vi "experiment control.vi"() -> ()   [LabVIEW 2012] (continued)
              tunnel: [w3762 w3766 w3770 w3775] -> w3734
              frame "A", Default {
                n1646 = Replace Array Subset(array=w3762, new element=TRUE ("new element/subarray"), index=w3765) -> (w3763:bool[])
              }
              frame "B" {
                n1647 = Replace Array Subset(array=w3766, new element=TRUE ("new element/subarray"), index=w3769) -> (w3767:bool[])
              }
              frame "C" {
                n1648 = Replace Array Subset(array=w3770, new element=TRUE ("new element/subarray"), index=w3773) -> (w3771:bool[])
              }
              frame "D" {
                n1649 = Replace Array Subset(array=w3774, new element=TRUE ("new element/subarray"), index=w3777) -> (w3775:bool[])
              }
            }
            n1650 = Bundle("Begin (ms)"=0.0, "Begin (ms)"=w3747, "DIO64 Line 4"=w3738, "DIO64 Line 4"=w3738, "DIO64 Line 4"=w3738, "DIO64 Line 4"=w3738) -> (w3749:T107)  [unwired: 1 in]
            n1651 = Bundle("Begin (ms)"=w3747, "Begin (ms)"=w3747, "DIO64 Line 4"=w3737, "DIO64 Line 4"=w3736, "DIO64 Line 4"=w3735, "DIO64 Line 4"=w3734) -> (w3752:T107)  [unwired: 1 in]
            n1652 = Bundle("Begin (ms)"=20.0, "Begin (ms)"=w3747, "DIO64 Line 4"=w3738, "DIO64 Line 4"=w3738, "DIO64 Line 4"=w3738, "DIO64 Line 4"=w3738) -> (w3748:T107)  [unwired: 1 in]
            n1653 = Build Array(w3749, w3752, w3748) -> (w3753:T108)
            n1654 = call "dt_i to 0-t_i.vi"("DIO64 Debug"=w3753) -> ("output cluster"=w3755:cluster{bool[][], bool[][], bool[][], bool[][]}, "DIOArray out 1"=w3756:bool[][], "ti"=w3757:dbl[])  [unwired: 2 in]
            n1655 = call "DIO64 Sequence.vi"("DIO64Addr (0)"=u16 0, "RepRate (Hz)"=10000.0, "Time Array (ms)"=w3757, "Set DIO line .."=w3756, "output cluster"=w3755, "error in"=w3760) -> ("error out"=w3759:errorcluster)  [unwired: 9 in]
          }
          frame "DIO64: Close" {
            n1656 = call "DIO64 Close.vi"("board in"=u16 0, "error in (no error)"=w3782) -> ("error out"=w3781:errorcluster)  [unwired: 12 in, 1 out]
            n1657 = Enqueue Element At Opposite End(queue=w3778, element="Debug: Console >> Closing DIO64") -> ()  [unwired: 2 in, 3 out]
          }
          frame "---------- Scope ----------" {
            # "Template Separator\n(You can make a copy of, or modify, this frame)"
          }
          frame "Scope: Initialise" {
            n1658 = case shown="\"TDS5034B\", Default" w3808 {
              tunnel: [w3812 w3814] -> w3795
              tunnel: ["SELect:CH4 ON" ("string") _] -> w3793
              tunnel: [w3812 w3814] -> w3791
              frame "TDS5034B", Default {
                n1659 = local read "TDS5034B Oscilloscope"() -> (w3812:T24)
              }
              frame "TDS2014" {
                n1660 = local read "TDS2014 Oscilloscope"() -> (w3814:T24)
              }
            }
            n1661 = Unbundle By Name(w3795) -> ("GPIB Address"=w3794:refnum<visa-resource-name>)
            n1662 = VISA Write(VISA resource name=w3794, write buffer="VERBOSE OFF" ("string"), error in (no error)=w3807) -> (VISA resource name out=w3802:refnum<visa-resource-name>, error out=w3803:errorcluster)  [unwired: 1 out]
            n1663 = VISA Write(VISA resource name=w3802, write buffer="HDR OFF" ("string"), error in (no error)=w3803) -> (VISA resource name out=w3801:refnum<visa-resource-name>, error out=w3800:errorcluster)  [unwired: 1 out]
            n1664 = VISA Write(VISA resource name=w3801, write buffer="DATA:ENC RIB" ("string"), error in (no error)=w3800) -> (VISA resource name out=w3796:refnum<visa-resource-name>, error out=w3797:errorcluster)  [unwired: 1 out]
            n1665 = VISA Write(VISA resource name=w3796, write buffer=w3793, error in (no error)=w3797) -> (error out=w3806:errorcluster)  [unwired: 2 out]
            n1666 = Unbundle By Name(w3806) -> ("status"=w3798:bool)  [unwired: 2 out]
            n1667 = Not(x=w3798) -> (.not. x?=w3792:bool)
            n1668 = Bundle By Name(cluster=w3791, "Detected"=w3792) -> (w3790:T24)
            n1669 = case shown="\"TDS5034B\", Default" w3808 {
              tunnel: w3790 -> [w3810 w3811]
              frame "TDS5034B", Default {
                n1670 = local write "TDS5034B Oscilloscope"(w3810) -> ()
              }
              frame "TDS2014" {
                n1671 = local write "TDS2014 Oscilloscope"(w3811) -> ()
              }
            }
            n1672 = Concatenate Strings("Debug: Console >> Initializing Scope ", w3808) -> (w3787:string)
            n1673 = Enqueue Element At Opposite End(queue=w3788, element=w3787) -> ()  [unwired: 2 in, 3 out]
          }
          frame "Scope: Start" {
            n1674 = case shown="\"TDS5034B\", Default" w3821 {
              tunnel: [w3853 w3854] -> w3818
              frame "TDS5034B", Default {
                n1675 = local read "TDS5034B Oscilloscope"() -> (w3853:T24)
              }
              frame "TDS2014" {
                n1676 = local read "TDS2014 Oscilloscope"() -> (w3854:T24)
              }
            }
            n1677 = Unbundle By Name(w3818) -> ("GPIB Address"=w3817:refnum<visa-resource-name>, "Detected"=w3816:bool)
            n1678 = case shown="True" w3816 {
              tunnel: w3820 -> [w3823 w3836]
              tunnel: w3817 -> [_ w3835]
              tunnel: [w3823 w3833] -> w3819
              frame False {
              }
              frame True {
                n1679 = VISA Write(VISA resource name=w3835, write buffer="Acq:State Stop" ("string"), error in (no error)=w3836) -> (VISA resource name out=w3824:refnum<visa-resource-name>, error out=w3825:errorcluster)  [unwired: 1 out]
                n1680 = VISA Write(VISA resource name=w3824, write buffer="ACQ:StopAfter Sequence" ("string"), error in (no error)=w3825) -> (VISA resource name out=w3832:refnum<visa-resource-name>, error out=w3831:errorcluster)  [unwired: 1 out]
                n1681 = VISA Write(VISA resource name=w3832, write buffer="ACQ:State Run" ("string"), error in (no error)=w3831) -> (error out=w3829:errorcluster)  [unwired: 2 out]
                n1682 = call "wait.vi"("error in (no error)"=w3829, "ms to wait"=u32 100) -> ("error out (no error)"=w3837:errorcluster)  [unwired: 7 in]
                n1683 = while {
                  tunnel: w3835 -> [w3847]
                  tunnel: w3837 -> [w3848]
                  tunnel: [w3846] -> w3834 mode=indexing
                  tunnel: [w3843] -> _
                  i -> [w3843]
                  stop <- w3840 stop-if-true
                  n1684 = VISA Write(VISA resource name=w3847, write buffer="Trig:State?", error in (no error)=w3848) -> (VISA resource name out=w3851:refnum<visa-resource-name>, error out=w3852:errorcluster)  [unwired: 1 out]
                  n1685 = VISA Read(VISA resource name=w3851, byte count=u32 50, error in (no error)=w3852) -> (read buffer=w3845:string, error out=w3846:errorcluster)  [unwired: 2 out]
                  n1686 = call <vilib>:"Trim Whitespace.vi"("string"=w3845) -> ("trimmed string"=w3841:string)  [unwired: 1 in]
                  n1687 = Equal?(x="REA" ("y"), y=w3841) -> (x = y?=w3839:bool)
                  n1688 = Equal?(x=w3841, y="SAV") -> (x = y?=w3838:bool)
                  n1689 = Or(x=w3839, y=w3838) -> (x .or. y?=w3840:bool)
                }
                n1690 = Merge Errors(w3834) -> (w3833:errorcluster)
              }
            }
          }
          frame "Scope: Read" {
            n1691 = case shown="\"TDS5034B\", Default" w3860 {
              tunnel: w3859 -> [w3866 w3899]
              tunnel: [w3864 w3897] -> w3858
              tunnel: w3857 -> [w3863 w3896]
              tunnel: [w3862 w3895] -> w3856
              frame "TDS5034B", Default {
                n1692 = local read "TDS5034B Oscilloscope"() -> (w3865:T24)
                n1693 = Unbundle By Name(w3865) -> ("GPIB Address"=w3868:refnum<visa-resource-name>, "Detected"=w3869:bool, "Channels"=w3867:u16[], "Resolution"=w3861:u16)
                n1694 = case shown="True" w3869 {
                  tunnel: w3868 -> [_ w3888]
                  tunnel: w3867 -> [_ w3887]
                  tunnel: w3866 -> [w3871 w3884]
                  tunnel: [w3871 w3882] -> w3864
                  tunnel: w3863 -> [w3870 w3880]
                  tunnel: [w3870 w3879] -> w3862
                  tunnel: w3861 -> [_ w3875]
                  frame False {
                  }
                  frame True {
                    n1695 = VISA Write(VISA resource name=w3888, write buffer="ACQ:State STOP", error in (no error)=w3884) -> (VISA resource name out=w3886:refnum<visa-resource-name>, error out=w3885:errorcluster)  [unwired: 1 out]
                    n1696 = for {
                      tunnel: w3887 -> [w3894] mode=indexing
                      tunnel: w3886 -> [w3893]
                      tunnel: w3885 -> [w3892]
                      tunnel: [w3891] -> w3883 mode=indexing
                      tunnel: [w3889] -> w3872 mode=indexing
                      n1697 = call "Fetch 5034B.vi"("error in (no error)"=w3892, "MaxTime (10000ms)"=u32 2000, "Ch (1=Ch1)"=w3894, "VISA resource name"=w3893) -> ("error out"=w3891:errorcluster, "Data Cluster"=w3889:cluster{"Y":dbl[], "t0":dbl, "dt":dbl})  [unwired: 4 in, 2 out]
                    }
                    n1698 = local write "TDS5034B Data"(w3872) -> ()
                    n1699 = Index Array(array=w3872) -> (element=w3878:cluster{"Y":dbl[], "t0":dbl, "dt":dbl})  [unwired: 1 in]
                    n1700 = Bundle By Name(cluster=w3880, "TDS5034B Data"=w3872) -> (w3879:T52)
                    n1701 = Unbundle By Name(w3878) -> ("Y"=w3877:dbl[])
                    n1702 = Merge Errors(w3883) -> (w3882:errorcluster)
                    n1703 = Array Size(array=w3877) -> (size(s)=w3876:i32)
                    "points" <- w3876
                    n1704 = To Double Precision Float(number=w3875) -> (double precision float=w3874:dbl)
                    n1705 = Divide(x=w3876, y=w3874) -> (x/y=→"frames":dbl)
                  }
                }
              }
              frame "TDS2014" {
                n1706 = local read "TDS2014 Oscilloscope"() -> (w3898:T24)
                n1707 = Unbundle By Name(w3898) -> ("GPIB Address"=w3901:refnum<visa-resource-name>, "Detected"=w3902:bool, "Channels"=w3900:u16[])
                n1708 = case shown="True" w3902 {
                  tunnel: w3901 -> [_ w3915]
                  tunnel: w3900 -> [_ w3914]
                  tunnel: w3899 -> [w3904 w3911]
                  tunnel: [w3904 w3909] -> w3897
                  tunnel: w3896 -> [w3903 w3907]
                  tunnel: [w3903 w3905] -> w3895
                  frame False {
                  }
                  frame True {
                    n1709 = VISA Write(VISA resource name=w3915, write buffer="ACQ:State STOP", error in (no error)=w3911) -> (VISA resource name out=w3913:refnum<visa-resource-name>, error out=w3912:errorcluster)  [unwired: 1 out]
                    n1710 = for {
                      tunnel: w3914 -> [w3921] mode=indexing
                      tunnel: w3913 -> [w3920]
                      tunnel: w3912 -> [w3919]
                      tunnel: [w3918] -> w3910 mode=indexing
                      tunnel: [w3916] -> w3906 mode=indexing
                      n1711 = call "Fetch 2014.vi"("error in (no error)"=w3919, "MaxTime (10000ms)"=u32 2000, "Ch (1=Ch1)"=w3921, "VISA resource name"=w3920) -> ("error out"=w3918:errorcluster, "Data Cluster"=w3916:cluster{"Y":dbl[], "t0":dbl, "dt":dbl})  [unwired: 4 in, 2 out]
                    }
                    n1712 = Bundle By Name(cluster=w3907, "TDS2014 Data"=w3906) -> (w3905:T52)
                    n1713 = Merge Errors(w3910) -> (w3909:errorcluster)
                  }
                }
              }
            }
          }
          frame "Scope: Settings" {
            n1714 = case shown="\"TDS5034B\", Default" w3925 {
              tunnel: w3924 -> [w3931 w3969]
              tunnel: [w3930 w3968] -> w3923
              frame "TDS5034B", Default {
                n1715 = local read "TDS5034B Oscilloscope"() -> (w3929:T24)
                n1716 = Unbundle By Name(w3929) -> ("GPIB Address"=w3932:refnum<visa-resource-name>, "Detected"=w3933:bool, "Resolution"=w3928:u16, "Frames"=w3927:u16)
                n1717 = case shown="True" w3933 {
                  tunnel: w3932 -> [_ w3964]
                  tunnel: w3931 -> [w3934 w3963]
                  tunnel: [w3934 w3945] -> w3930
                  tunnel: w3928 -> [_ w3955]
                  tunnel: w3929 -> [_ w3942]
                  tunnel: w3927 -> [_ w3940]
                  frame False {
                  }
                  frame True {
                    n1718 = Number To Decimal String(number=w3955) -> (decimal integer string=w3952:string)  [unwired: 1 in]
                    n1719 = Number To Decimal String(number=w3940) -> (decimal integer string=w3947:string)  [unwired: 1 in]
                    n1720 = Concatenate Strings("Hor:Reso " ("write buffer"), w3952) -> (w3953:string)
                    n1721 = Concatenate Strings("Hor:Fast:Len " ("write buffer"), w3952) -> (w3950:string)
                    n1722 = Concatenate Strings("Hor:Fast:Count " ("write buffer"), w3947) -> (w3948:string)
                    n1723 = VISA Write(VISA resource name=w3964, write buffer=w3953, error in (no error)=w3963) -> (VISA resource name out=w3961:refnum<visa-resource-name>, error out=w3962:errorcluster)  [unwired: 1 out]
                    n1724 = VISA Write(VISA resource name=w3961, write buffer="Hor:Fast:State On", error in (no error)=w3962) -> (VISA resource name out=w3959:refnum<visa-resource-name>, error out=w3960:errorcluster)  [unwired: 1 out]
                    n1725 = VISA Write(VISA resource name=w3959, write buffer=w3950, error in (no error)=w3960) -> (VISA resource name out=w3957:refnum<visa-resource-name>, error out=w3958:errorcluster)  [unwired: 1 out]
                    n1726 = VISA Write(VISA resource name=w3957, write buffer=w3948, error in (no error)=w3958) -> (VISA resource name out=w3936:refnum<visa-resource-name>, error out=w3935:errorcluster)  [unwired: 1 out]
                    n1727 = VISA Write(VISA resource name=w3936, write buffer="Hor:Reso?", error in (no error)=w3935) -> (VISA resource name out=w3939:refnum<visa-resource-name>, error out=w3938:errorcluster)  [unwired: 1 out]
                    n1728 = VISA Read(VISA resource name=w3939, byte count=u32 50, error in (no error)=w3938) -> (read buffer=w3944:string, error out=w3945:errorcluster)  [unwired: 2 out]
                    n1729 = Decimal String To Number(string=w3944) -> (number=w3943:i32)  [unwired: 2 in, 1 out]
                    n1730 = Bundle By Name(cluster=w3942, "Resolution"=w3943) -> (w3941:T24)
                    n1731 = local write "TDS5034B Oscilloscope"(w3941) -> ()
                  }
                }
              }
              frame "TDS2014" {
                n1732 = local read "TDS2014 Oscilloscope"() -> (w3967:T24)
                n1733 = Unbundle By Name(w3967) -> ("GPIB Address"=w3970:refnum<visa-resource-name>, "Detected"=w3971:bool, "Resolution"=w3966:u16, "Frames"=w3965:u16)
                n1734 = case shown="True" w3971 {
                  tunnel: w3970 -> [_ w3981]
                  tunnel: w3969 -> [w3972 w3982]
                  tunnel: [w3972 w3999] -> w3968
                  tunnel: w3966 -> [_ _]
                  tunnel: w3967 -> [_ w3996]
                  tunnel: w3965 -> [_ w3978]
                  frame False {
                  }
                  frame True {
                    n1735 = Number To Decimal String(number=w3978) -> (decimal integer string=w3979:string)  [unwired: 1 in]
                    n1736 = Concatenate Strings("Acq:NumAv" ("write buffer"), w3979) -> (w3977:string)
                    n1737 = VISA Write(VISA resource name=w3981, write buffer="Acq:Mode SAM", error in (no error)=w3982) -> (VISA resource name out=w3991:refnum<visa-resource-name>, error out=w3983:errorcluster)  [unwired: 1 out]
                    n1738 = VISA Write(VISA resource name=w3991, write buffer=w3977, error in (no error)=w3983) -> (VISA resource name out=w3984:refnum<visa-resource-name>, error out=w3985:errorcluster)  [unwired: 1 out]
                    n1739 = VISA Write(VISA resource name=w3984, write buffer="Acq:NumAv?", error in (no error)=w3985) -> (VISA resource name out=w3974:refnum<visa-resource-name>, error out=w3975:errorcluster)  [unwired: 1 out]
                    n1740 = VISA Read(VISA resource name=w3974, byte count=u32 50, error in (no error)=w3975) -> (VISA resource name out=w3986:refnum<visa-resource-name>, read buffer=w3989:string, error out=w3987:errorcluster)  [unwired: 1 out]
                    n1741 = VISA Write(VISA resource name=w3986, write buffer="Hor:Reco?", error in (no error)=w3987) -> (VISA resource name out=w3994:refnum<visa-resource-name>, error out=w3993:errorcluster)  [unwired: 1 out]
                    n1742 = VISA Read(VISA resource name=w3994, byte count=u32 50, error in (no error)=w3993) -> (read buffer=w3998:string, error out=w3999:errorcluster)  [unwired: 2 out]
                    n1743 = Decimal String To Number(string=w3998) -> (number=w3997:i32)  [unwired: 2 in, 1 out]
                    n1744 = Decimal String To Number(string=w3989) -> (number=w3990:i32)  [unwired: 2 in, 1 out]
                    n1745 = Bundle By Name(cluster=w3996, "Resolution"=w3997, "Frames"=w3990) -> (w3995:T24)
                    n1746 = local write "TDS2014 Oscilloscope"(w3995) -> ()
                  }
                }
              }
            }
          }
          frame "Scope: Trigger Settings" {
            n1747 = case shown="\"TDS5034B\", Default" w4004 {
              tunnel: w4003 -> [w4010 w4051]
              tunnel: [w4009 w4050] -> w4002
              frame "TDS5034B", Default {
                n1748 = local read "TDS5034B Oscilloscope"() -> (w4008:T24)
                n1749 = Unbundle By Name(w4008) -> ("GPIB Address"=w4011:refnum<visa-resource-name>, "Detected"=w4012:bool, "Trigger Position"=w4007:dbl, "Trigger Level"=w4006:dbl)
                n1750 = case shown="True" w4012 {
                  tunnel: w4011 -> [_ w4031]
                  tunnel: w4010 -> [w4013 w4032]
                  tunnel: [w4013 w4022] -> w4009
                  tunnel: w4008 -> [_ w4041]
                  tunnel: w4007 -> [_ w4037]
                  tunnel: w4006 -> [_ w4028]
                  frame False {
                  }
                  frame True {
                    n1751 = Number To Engineering String(4:w4037) -> (0:w4038:string)  [unwired: 3 in]
                    n1752 = Number To Engineering String(4:w4028) -> (0:w4030:string)  [unwired: 3 in]
                    n1753 = Concatenate Strings("Hor:Pos " ("write buffer"), w4038) -> (w4034:string)
                    n1754 = Concatenate Strings("Trig:A:Lev " ("write buffer"), w4030) -> (w4018:string)
                    n1755 = VISA Write(VISA resource name=w4031, write buffer=w4034, error in (no error)=w4032) -> (VISA resource name out=w4036:refnum<visa-resource-name>, error out=w4035:errorcluster)  [unwired: 1 out]
                    n1756 = VISA Write(VISA resource name=w4036, write buffer="Hor:Pos?", error in (no error)=w4035) -> (VISA resource name out=w4026:refnum<visa-resource-name>, error out=w4025:errorcluster)  [unwired: 1 out]
                    n1757 = VISA Read(VISA resource name=w4026, byte count=u32 50, error in (no error)=w4025) -> (VISA resource name out=w4015:refnum<visa-resource-name>, read buffer=w4043:string, error out=w4017:errorcluster)  [unwired: 1 out]
                    n1758 = Fract/Exp String To Number(string=w4043) -> (number=w4042:dbl)  [unwired: 3 in, 1 out]
                    n1759 = VISA Write(VISA resource name=w4015, write buffer=w4018, error in (no error)=w4017) -> (VISA resource name out=w4014:refnum<visa-resource-name>, error out=w4016:errorcluster)  [unwired: 1 out]
                    n1760 = VISA Write(VISA resource name=w4014, write buffer="Trig:A:Lev?", error in (no error)=w4016) -> (VISA resource name out=w4023:refnum<visa-resource-name>, error out=w4021:errorcluster)  [unwired: 1 out]
                    n1761 = VISA Read(VISA resource name=w4023, byte count=u32 50, error in (no error)=w4021) -> (read buffer=w4024:string, error out=w4022:errorcluster)  [unwired: 2 out]
                    n1762 = Fract/Exp String To Number(string=w4024) -> (number=w4019:dbl)  [unwired: 3 in, 1 out]
                    n1763 = Bundle By Name(cluster=w4041, "Trigger Position"=w4042, "Trigger Level"=w4019) -> (w4040:T24)
                    n1764 = local write "TDS5034B Oscilloscope"(w4040) -> ()
                  }
                }
              }
              frame "TDS2014" {
                n1765 = local read "TDS2014 Oscilloscope"() -> (w4049:T24)
                n1766 = Unbundle By Name(w4049) -> ("GPIB Address"=w4052:refnum<visa-resource-name>, "Detected"=w4053:bool, "Trigger Position"=w4047:dbl, "Trigger Level"=w4048:dbl)
                n1767 = Divide(x=w4047, y=1000.0) -> (x/y=w4045:dbl)
                n1768 = case shown="True" w4053 {
                  tunnel: w4052 -> [_ w4075]
                  tunnel: w4051 -> [w4054 w4076]
                  tunnel: [w4054 w4066] -> w4050
                  tunnel: w4049 -> [_ w4085]
                  tunnel: w4045 -> [_ w4081]
                  tunnel: w4048 -> [_ w4072]
                  frame False {
                  }
                  frame True {
                    n1769 = Number To Engineering String(4:w4081) -> (0:w4082:string)  [unwired: 3 in]
                    n1770 = Number To Engineering String(4:w4072) -> (0:w4074:string)  [unwired: 3 in]
                    n1771 = Concatenate Strings("Hor:Pos " ("write buffer"), w4082) -> (w4078:string)
                    n1772 = Concatenate Strings("Trig:MAI:Lev " ("write buffer"), w4074) -> (w4062:string)
                    n1773 = VISA Write(VISA resource name=w4075, write buffer=w4078, error in (no error)=w4076) -> (VISA resource name out=w4080:refnum<visa-resource-name>, error out=w4079:errorcluster)  [unwired: 1 out]
                    n1774 = VISA Write(VISA resource name=w4080, write buffer="Hor:Pos?", error in (no error)=w4079) -> (VISA resource name out=w4070:refnum<visa-resource-name>, error out=w4069:errorcluster)  [unwired: 1 out]
                    n1775 = VISA Read(VISA resource name=w4070, byte count=u32 50, error in (no error)=w4069) -> (VISA resource name out=w4059:refnum<visa-resource-name>, read buffer=w4086:string, error out=w4061:errorcluster)  [unwired: 1 out]
                    n1776 = Fract/Exp String To Number(string=w4086) -> (number=w4056:dbl)  [unwired: 3 in, 1 out]
                    n1777 = VISA Write(VISA resource name=w4059, write buffer=w4062, error in (no error)=w4061) -> (VISA resource name out=w4058:refnum<visa-resource-name>, error out=w4060:errorcluster)  [unwired: 1 out]
                    n1778 = VISA Write(VISA resource name=w4058, write buffer="Trig:MAI:Lev?", error in (no error)=w4060) -> (VISA resource name out=w4067:refnum<visa-resource-name>, error out=w4065:errorcluster)  [unwired: 1 out]
                    n1779 = Multiply(x=w4056, y=1000.0) -> (x*y=w4055:dbl)
                    n1780 = VISA Read(VISA resource name=w4067, byte count=u32 50, error in (no error)=w4065) -> (read buffer=w4068:string, error out=w4066:errorcluster)  [unwired: 2 out]
                    n1781 = Fract/Exp String To Number(string=w4068) -> (number=w4063:dbl)  [unwired: 3 in, 1 out]
                    n1782 = Bundle By Name(cluster=w4085, "Trigger Position"=w4055, "Trigger Level"=w4063) -> (w4084:T24)
                    n1783 = local write "TDS2014 Oscilloscope"(w4084) -> ()
                  }
                }
              }
            }
          }
          frame "Scope: Measurement Settings" {
            n1784 = case shown="\"TDS2014\", Default" w4091 {
              tunnel: w4090 -> [w4096]
              tunnel: [w4095] -> w4089
              frame "TDS2014", Default {
                n1785 = local read "TDS2014 Oscilloscope"() -> (w4094:T24)
                n1786 = Unbundle By Name(w4094) -> ("GPIB Address"=w4097:refnum<visa-resource-name>, "Detected"=w4098:bool, "Measurements"=w4093:T109)
                n1787 = case shown="True" w4098 {
                  tunnel: w4097 -> [_ w4101]
                  tunnel: w4096 -> [w4099 w4102]
                  tunnel: [w4099 w4100] -> w4095
                  tunnel: w4094 -> [_ _]
                  tunnel: w4093 -> [_ w4103]
                  frame False {
                  }
                  frame True {
                    n1788 = for {
                      tunnel: w4103 -> [w4119] mode=indexing
                      shift-right: [w4107] -> w4100
                      shift-left: w4102 -> [w4120]
                      shift-right: [w4106] -> _
                      shift-left: w4101 -> [w4121]
                      i -> [w4105]
                      n1789 = Increment(x=w4105) -> (x+1=w4104:i32)
                      n1790 = Unbundle By Name(w4119) -> ("Source"=w4110:string, "Type"=w4109:string)
                      n1791 = Number To Decimal String(number=w4104) -> (decimal integer string=w4108:string)  [unwired: 1 in]
                      n1792 = Concatenate Strings("Measu:Meas", w4108, ":Source ", w4110) -> (w4117:string)
                      n1793 = VISA Write(VISA resource name=w4121, write buffer=w4117, error in (no error)=w4120) -> (VISA resource name out=w4112:refnum<visa-resource-name>, error out=w4113:errorcluster)  [unwired: 1 out]
                      n1794 = Concatenate Strings("Measu:Meas", w4108, ":Type ", w4109) -> (w4111:string)
                      n1795 = VISA Write(VISA resource name=w4112, write buffer=w4111, error in (no error)=w4113) -> (VISA resource name out=w4106:refnum<visa-resource-name>, error out=w4107:errorcluster)  [unwired: 1 out]
                    }
                  }
                }
              }
            }
          }
          frame "Scope: Measurement" {
            n1796 = case shown="\"TDS2014\", Default" w4125 {
              tunnel: w4124 -> [w4130]
              tunnel: [w4129] -> w4123
              frame "TDS2014", Default {
                n1797 = local read "TDS2014 Oscilloscope"() -> (w4128:T24)
                n1798 = Unbundle By Name(w4128) -> ("GPIB Address"=w4131:refnum<visa-resource-name>, "Detected"=w4132:bool, "Measurements"=w4127:T109)
                n1799 = case shown="True" w4132 {
                  tunnel: w4131 -> [_ w4138]
                  tunnel: w4130 -> [w4133 w4139]
                  tunnel: [w4133 w4137] -> w4129
                  tunnel: w4128 -> [_ w4135]
                  tunnel: w4127 -> [_ w4140]
                  frame False {
                  }
                  frame True {
                    n1800 = for {
                      tunnel: w4140 -> [w4145] mode=indexing
                      shift-right: [w4149] -> w4137
                      shift-left: w4139 -> [w4156]
                      shift-right: [w4148] -> _
                      shift-left: w4138 -> [w4157]
                      tunnel: [w4143] -> w4136 mode=indexing
                      i -> [w4142]
                      n1801 = Increment(x=w4142) -> (x+1=w4141:i32)
                      n1802 = Number To Decimal String(number=w4141) -> (decimal integer string=w4150:string)  [unwired: 1 in]
                      n1803 = Concatenate Strings("Measu:Meas", w4150, ":Value? ") -> (w4154:string)
                      n1804 = VISA Write(VISA resource name=w4157, write buffer=w4154, error in (no error)=w4156) -> (VISA resource name out=w4151:refnum<visa-resource-name>, error out=w4152:errorcluster)  [unwired: 1 out]
                      n1805 = VISA Read(VISA resource name=w4151, byte count=u32 50, error in (no error)=w4152) -> (VISA resource name out=w4148:refnum<visa-resource-name>, read buffer=w4146:string, error out=w4149:errorcluster)  [unwired: 1 out]
                      n1806 = Fract/Exp String To Number(string=w4146) -> (number=w4144:dbl)  [unwired: 3 in, 1 out]
                      n1807 = Bundle By Name(cluster=w4145, "Value"=w4144) -> (w4143:T110)
                    }
                    n1808 = Bundle By Name(cluster=w4135, "Measurements"=w4136) -> (w4134:T24)
                    n1809 = local write "TDS2014 Oscilloscope"(w4134) -> ()
                  }
                }
              }
            }
          }
          frame "Scope: Display Traces" {
            n1810 = case shown="\"TDS5034B\", Default" w4161 {
              tunnel: w4159 -> [w4164 w4231]
              frame "TDS5034B", Default {
                n1811 = local read "TDS5034B Oscilloscope"() -> (w4163:T24)
                n1812 = Unbundle By Name(w4163) -> ("Detected"=w4162:bool)
                n1813 = case shown="True" w4162 {
                  tunnel: w4164 -> [_ w4169]
                  tunnel: w4163 -> [_ w4165]
                  frame False {
                  }
                  frame True {
                    w4172 = 10.0 ("y value")
                    n1814 = local read "Frames and Rep Rate"() -> (w4167:cluster{"Frames":i32, "Repetition Rate":dbl})
                    n1815 = Unbundle By Name(w4169) -> ("TDS5034B Data"=w4168:cluster{"Y":dbl[], "t0":dbl, "dt":dbl}[])
                    n1816 = Unbundle By Name(w4167) -> ("Frames"=w4166:i32)
                    n1817 = property on="Channel" class="Ring (strict)"() -> ("StringsAndValues[]"=w4179:T111)  [unwired: 2 in, 2 out]
                    n1818 = Unbundle By Name(w4165) -> ("Channels"=w4181:u16[])
                    n1819 = for {
                      tunnel: w4168 -> [w4225] mode=indexing
                      tunnel: [w4224] -> w4182 mode=indexing
                      tunnel: w4166 -> [w4214]
                      n1820 = Unbundle By Name(w4225) -> ("Y"=w4217:dbl[], "dt"=w4218:dbl)
                      n1821 = Array Size(array=w4217) -> (size(s)=w4216:i32)
                      n1822 = Divide(x=w4216, y=w4214) -> (x/y=w4215:dbl)
                      n1823 = Reshape Array(w4217, w4214, w4215) -> (w4222:dbl[][])
                      n1824 = Transpose 2D Array(2D array=w4222) -> (transposed array=w4223:dbl[][])
                      n1825 = for {
                        tunnel: w4223 -> [w4229] mode=indexing
                        tunnel: [w4227] -> w4221 mode=indexing
                        tunnel: w4214 -> [w4226]
                        n1826 = Add Array Elements(numeric array=w4229) -> (sum=w4228:dbl)
                        n1827 = Divide(x=w4228, y=w4226) -> (x/y=w4227:dbl)
                      }
                      n1828 = Select(t=w4221, s=TRUE, f=w4217) -> (s? t:f=w4219:dbl[])
                      n1829 = Bundle By Name("Y"=w4219, "dt"=w4218) -> (w4224:waveform(dbl))  [unwired: 1 in]
                    }
                    n1830 = Array Size(array=w4181) -> (size(s)=w4180:i32)
                    n1831 = for {
                      tunnel: w4179 -> [w4208] mode=indexing
                      tunnel: [w4207] -> w4178 mode=indexing
                      tunnel: [w4206] -> w4177 mode=indexing
                      n1832 = Unbundle By Name(w4208) -> ("Value"=w4207:u16, "String"=w4206:string)
                    }
                    n1833 = property on="Waveform Chart" class="WFChart (strict)"("LegNumRows"=w4180) -> ()  [unwired: 2 in, 2 out]
                    n1834 = for {
                      tunnel: w4181 -> [w4212] mode=indexing
                      tunnel: w4178 -> [w4213]
                      tunnel: w4177 -> [w4211]
                      tunnel: [w4209] -> w4176 mode=indexing
                      n1835 = Search 1D Array(1D array=w4213, element=w4212) -> (index of element=w4210:i32)  [unwired: 1 in]
                      n1836 = Index Array(array=w4211, index=w4210) -> (element=w4209:string)
                    }
                    n1837 = for {
                      tunnel: w4176 -> [w4199] mode=indexing
                      i -> [w4198]
                      n1838 = stacked-sequence {
                        tunnel: w4199 -> [_ w4201]
                        tunnel: w4198 -> [w4200 _]
                        frame #0 {
                          n1839 = property on="Waveform Chart" class="WFChart (strict)"("Active Plot"=w4200) -> ()  [unwired: 2 in, 2 out]
                        }
                        frame #1 {
                          n1840 = case shown="\"Channel 1\"" w4201 {
                            frame Default {
                            }
                            frame "Channel 1" {
                              n1841 = property on="Waveform Chart" class="WFChart (strict)"("Plot.Plot Color"=u32 16776960) -> ()  [unwired: 2 in, 2 out]
                            }
                            frame "Channel 2" {
                              n1842 = property on="Waveform Chart" class="WFChart (strict)"("Plot.Plot Color"=u32 51455) -> ()  [unwired: 2 in, 2 out]
                            }
                            frame "Channel 3" {
                              n1843 = property on="Waveform Chart" class="WFChart (strict)"("Plot.Plot Color"=u32 15566272) -> ()  [unwired: 2 in, 2 out]
                            }
                            frame "Channel 4" {
                              n1844 = property on="Waveform Chart" class="WFChart (strict)"("Plot.Plot Color"=u32 2555802) -> ()  [unwired: 2 in, 2 out]
                            }
                          }
                          n1845 = property on="Waveform Chart" class="WFChart (strict)"("Plot.Plot Name"=w4201) -> ()  [unwired: 2 in, 2 out]
                        }
                      }
                    }
                    n1846 = stacked-sequence {
                      seq-local: [w4185 _ _] -> [_ w4188 _]
                      seq-local: [w4183 _ _] -> [_ w4187 _]
                      seq-local: [w4184 _ _] -> [_ w4186 _]
                      seq-local: [_ w4187 _] -> [_ _ w4189]
                      seq-local: [_ w4186 _] -> [_ _ w4190]
                      tunnel: w4182 -> [w4185 _ _]
                      tunnel: [_ _ w4189] -> w4170
                      frame #0 {
                        n1847 = property on="Waveform Chart" class="WFChart (strict)"() -> ("XScale.Range"=w4183:T112, "YScale.Range"=w4184:T112)  [unwired: 2 in, 2 out]
                      }
                      frame #1 {
                        n1848 = local write "Waveform Chart"(w4188) -> ()
                      }
                      frame #2 {
                        n1849 = disable-structure shown="Disabled" {
                          disable-tunnel: w4190 -> [w4192 _]
                          disable-tunnel: w4189 -> [w4191 _]
                          frame Disabled {
                            n1850 = property on="Waveform Chart" class="WFChart (strict)"("XScale.Range"=w4191, "YScale.Range"=w4192) -> ()  [unwired: 2 in, 2 out]
                          }
                          frame Enabled {
                          }
                        }
                      }
                    }
                    n1851 = Unbundle By Name(w4170) -> ("Maximum"=w4175:dbl, "Minimum"=w4174:dbl)
                    n1852 = Build Array(w4175, w4174) -> (w4173:dbl[])
                    n1853 = for {
                      N: w4172 -> [_]
                      tunnel: w4173 -> [w4197]
                      tunnel: w4172 -> [w4194]
                      tunnel: [w4193] -> w4171 mode=indexing
                      i -> [w4196]
                      n1854 = Divide(x=w4196, y=w4194) -> (x/y=w4195:dbl)
                      n1855 = Interpolate 1D Array(1:w4195, 2:w4197) -> (0:w4193:dbl)
                    }
                    n1856 = property on="Waveform Chart" class="WFChart (strict)"("XScale.MarkerVals[]"=w4171) -> ()  [unwired: 2 in, 2 out]
                  }
                }
              }
              frame "TDS2014" {
                w4234 = 10.0 ("y value")
                n1857 = local read "TDS2014 Oscilloscope"() -> (w4253:T24)
                n1858 = Unbundle By Name(w4231) -> ("TDS2014 Data"=w4230:cluster{"Y":dbl[], "t0":dbl, "dt":dbl}[])
                n1859 = Unbundle By Name(w4253) -> ("Frames"=w4249:u16, "Resolution"=w4248:u16, "Frames"=w4247:u16, "Channels"=w4251:u16[])
                n1860 = property on="Channel" class="Ring (strict)"() -> ("StringsAndValues[]"=w4246:T111)  [unwired: 2 in, 2 out]
                n1861 = for {
                  tunnel: w4230 -> [w4296] mode=indexing
                  tunnel: [w4295] -> w4252 mode=indexing
                  tunnel: w4249 -> [w4290]
                  tunnel: w4248 -> [w4289]
                  tunnel: w4247 -> [w4287]
                  n1862 = Unbundle By Name(w4296) -> ("Y"=w4292:dbl[], "dt"=w4285:dbl)
                  n1863 = Reshape Array(w4292, w4290, w4289) -> (w4293:dbl[][])
                  n1864 = Transpose 2D Array(2D array=w4293) -> (transposed array=w4294:dbl[][])
                  n1865 = for {
                    tunnel: w4294 -> [w4300] mode=indexing
                    tunnel: [w4298] -> w4291 mode=indexing
                    tunnel: w4287 -> [w4297]
                    n1866 = Add Array Elements(numeric array=w4300) -> (sum=w4299:dbl)
                    n1867 = Divide(x=w4299, y=w4297) -> (x/y=w4298:dbl)
                  }
                  n1868 = Select(t=w4291, s=TRUE, f=w4292) -> (s? t:f=w4286:dbl[])
                  n1869 = Bundle By Name("Y"=w4286, "dt"=w4285) -> (w4295:waveform(dbl))  [unwired: 1 in]
                }
                n1870 = Array Size(array=w4251) -> (size(s)=w4250:i32)
                n1871 = for {
                  tunnel: w4246 -> [w4279] mode=indexing
                  tunnel: [w4278] -> w4245 mode=indexing
                  tunnel: [w4277] -> w4244 mode=indexing
                  n1872 = Unbundle By Name(w4279) -> ("Value"=w4278:u16, "String"=w4277:string)
                }
                n1873 = property on="Waveform Chart" class="WFChart (strict)"("LegNumRows"=w4250) -> ()  [unwired: 2 in, 2 out]
                n1874 = for {
                  tunnel: w4251 -> [w4283] mode=indexing
                  tunnel: w4245 -> [w4284]
                  tunnel: w4244 -> [w4282]
                  tunnel: [w4280] -> w4243 mode=indexing
                  n1875 = Search 1D Array(1D array=w4284, element=w4283) -> (index of element=w4281:i32)  [unwired: 1 in]
                  n1876 = Index Array(array=w4282, index=w4281) -> (element=w4280:string)
                }
                n1877 = for {
                  tunnel: w4243 -> [w4270] mode=indexing
                  i -> [w4269]
                  n1878 = stacked-sequence {
                    tunnel: w4270 -> [_ w4272]
                    tunnel: w4269 -> [w4271 _]
                    frame #0 {
                      n1879 = property on="Waveform Chart" class="WFChart (strict)"("Active Plot"=w4271) -> ()  [unwired: 2 in, 2 out]
                    }
                    frame #1 {
                      n1880 = case shown="\"Channel 1\"" w4272 {
                        frame Default {
                        }
                        frame "Channel 1" {
                          n1881 = property on="Waveform Chart" class="WFChart (strict)"("Plot.Plot Color"=u32 16776960) -> ()  [unwired: 2 in, 2 out]
                        }
                        frame "Channel 2" {
                          n1882 = property on="Waveform Chart" class="WFChart (strict)"("Plot.Plot Color"=u32 51455) -> ()  [unwired: 2 in, 2 out]
                        }
                        frame "Channel 3" {
                          n1883 = property on="Waveform Chart" class="WFChart (strict)"("Plot.Plot Color"=u32 15566272) -> ()  [unwired: 2 in, 2 out]
                        }
                        frame "Channel 4" {
                          n1884 = property on="Waveform Chart" class="WFChart (strict)"("Plot.Plot Color"=u32 2555802) -> ()  [unwired: 2 in, 2 out]
                        }
                      }
                      n1885 = property on="Waveform Chart" class="WFChart (strict)"("Plot.Plot Name"=w4272) -> ()  [unwired: 2 in, 2 out]
                    }
                  }
                }
                n1886 = Unbundle By Name(w4232) -> ("Maximum"=w4237:dbl, "Minimum"=w4236:dbl)
                n1887 = Build Array(w4237, w4236) -> (w4235:dbl[])
                n1888 = for {
                  N: w4234 -> [_]
                  tunnel: w4235 -> [w4258]
                  tunnel: w4234 -> [w4255]
                  tunnel: [w4254] -> w4233 mode=indexing
                  i -> [w4257]
                  n1889 = Divide(x=w4257, y=w4255) -> (x/y=w4256:dbl)
                  n1890 = Interpolate 1D Array(1:w4256, 2:w4258) -> (0:w4254:dbl)
                }
                n1891 = flat-sequence {
                  tunnel: w4252 -> [w4261]
                  tunnel: [w4261] -> w4242
                  tunnel: [w4259] -> w4240
                  tunnel: [w4260] -> w4239
                  tunnel: w4242 -> [w4264]
                  tunnel: [w4263] -> w4241
                  tunnel: w4240 -> [w4263]
                  tunnel: w4239 -> [w4262]
                  tunnel: [w4262] -> w4238
                  tunnel: w4241 -> [w4265]
                  tunnel: w4238 -> [w4266]
                  tunnel: [w4265] -> w4232
                  frame #0 {
                    n1892 = property on="Waveform Chart" class="WFChart (strict)"() -> ("XScale.Range"=w4259:T112, "YScale.Range"=w4260:T112)  [unwired: 2 in, 2 out]
                  }
                  frame #1 {
                    n1893 = local write "Waveform Chart"(w4264) -> ()
                  }
                  frame #2 {
                    n1894 = disable-structure shown="Disabled" {
                      disable-tunnel: w4266 -> [w4268 _]
                      disable-tunnel: w4265 -> [w4267 _]
                      frame Disabled {
                        n1895 = property on="Waveform Chart" class="WFChart (strict)"("XScale.Range"=w4267, "YScale.Range"=w4268) -> ()  [unwired: 2 in, 2 out]
                      }
                      frame Enabled {
                      }
                    }
                  }
                }
                n1896 = property on="Waveform Chart" class="WFChart (strict)"("XScale.MarkerVals[]"=w4233) -> ()  [unwired: 2 in, 2 out]
              }
            }
          }
          frame "Scope: Stop" {
            n1897 = case shown="\"TDS5034B\", Default" w4307 {
              tunnel: [w4314 w4315] -> w4303
              frame "TDS5034B", Default {
                n1898 = local read "TDS5034B Oscilloscope"() -> (w4314:T24)
              }
              frame "TDS2014" {
                n1899 = local read "TDS2014 Oscilloscope"() -> (w4315:T24)
              }
            }
            n1900 = Unbundle By Name(w4303) -> ("GPIB Address"=w4302:refnum<visa-resource-name>, "Detected"=w4301:bool)
            n1901 = case shown="True" w4301 {
              tunnel: w4306 -> [w4309 w4312]
              tunnel: w4302 -> [_ w4311]
              tunnel: [w4309 w4310] -> w4305
              frame False {
              }
              frame True {
                n1902 = VISA Write(VISA resource name=w4311, write buffer="ACQ:State STOP" ("string"), error in (no error)=w4312) -> (error out=w4310:errorcluster)  [unwired: 2 out]
              }
            }
          }
          frame "Scope: Close" {
            n1903 = case shown="\"TDS5034B\", Default" w4322 {
              tunnel: [w4328 w4329] -> w4318
              frame "TDS5034B", Default {
                n1904 = local read "TDS5034B Oscilloscope"() -> (w4328:T24)
              }
              frame "TDS2014" {
                n1905 = local read "TDS2014 Oscilloscope"() -> (w4329:T24)
              }
            }
            n1906 = Unbundle By Name(w4318) -> ("GPIB Address"=w4317:refnum<visa-resource-name>, "Detected"=w4316:bool)
            n1907 = case shown="True" w4316 {
              tunnel: w4321 -> [w4324 w4326]
              tunnel: w4317 -> [_ w4327]
              tunnel: [w4324 w4325] -> w4320
              frame False {
              }
              frame True {
                n1908 = VISA Close(VISA resource name=w4327, error in (no error)=w4326) -> (error out=w4325:errorcluster)
              }
            }
          }
          frame "---------- DDS ----------" {
            # "Template Separator\n(You can make a copy of, or modify, this frame)"
          }
          frame "Trap DDS: Set Clock" {
            w4335 = FALSE ("VCO Gain")
            n1909 = local read "Trap DDS"() -> (w4340:T26)
            n1910 = Unbundle By Name(w4340) -> ("usb 1"=w4341:refnum<visa-resource-name>, "usb 2"=w4337:refnum<visa-resource-name>, "pll multiplier"=w4336:u8)
            n1911 = call "DDS9959 Set Clock.vi"("error in (no error)"=w4344, "VCO Gain"=w4335, "PLL Multiplier"=w4336, "VISA resource name"=w4341) -> ("error out"=w4334:errorcluster)  [unwired: 6 in, 1 out]
            n1912 = call "DDS9959 Set Clock.vi"("error in (no error)"=w4334, "VCO Gain"=w4335, "PLL Multiplier"=w4336, "VISA resource name"=w4337) -> ("error out"=w4343:errorcluster)  [unwired: 6 in, 1 out]
            n1913 = Unbundle By Name(w4343) -> ("status"=w4339:bool)
